vi "Get Displayed Tree Items.vi"(10 "Displayed Items":string[](array[string]), 11 "TreeItems":T1[](array[typedef])) -> (2 "TreeItem Indices (Displayed Items)":i32[](array[numeric]), 3 "TreeItems (duplicate)":T1[](array[typedef]))   [LabVIEW 2020, in "BetterDragAndDrop.lvlib" / "BetterTreeHandle.lvclass"]
uses:
  Classes/BetterTreeHandle/BetterTreeHandle.lvclass
  Classes/BetterTreeItem/SubVIs/TreeItem.ctl
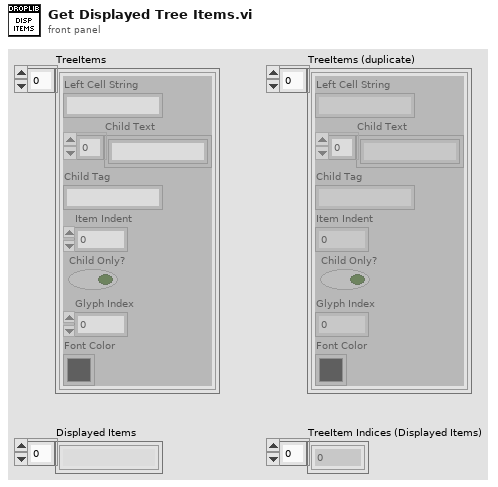
[diagram p1: front panel]
types:
  T1 = typedef "BetterDragAndDrop.lvlib/BetterTreeHandle.lvclass/TreeItem.ctl" = cluster{"Left Cell String":string, "Child Text":string[], "Child Tag":string, "Item Indent":i32, "Child Only?":bool, "Glyph Index":i32, "Font Color":u32}
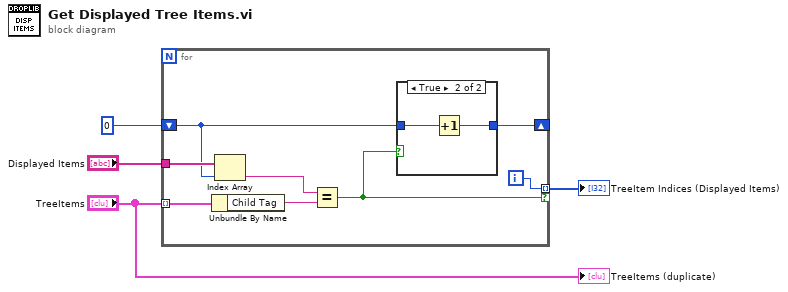
[diagram p0: block diagram]
diagram:
  n1 = for {
    tunnel: "Displayed Items" -> [w11]
    tunnel: [w5] -> w1 mode=indexing if=w8
    tunnel: "TreeItems" -> [w12] mode=indexing
    shift-right: [w6] -> _
    shift-left: 0 -> [w7]
    i -> [w5]
    n2 = Unbundle By Name(w12) -> ("Child Tag"=w10:string)
    n3 = Index Array(array=w11, index=w7) -> (element=w9:string)
    n4 = Equal?(x=w9, y=w10) -> (x = y?=w8:bool)
    n5 = case shown="True" w8 {
      tunnel: w7 -> [w13 w15]
      tunnel: [w13 w14] -> w6
      frame False {
      }
      frame True {
        n6 = Increment(x=w15) -> (x+1=w14:i32)
      }
    }
  }
  "TreeItem Indices (Displayed Items)" <- w1
  "TreeItems (duplicate)" <- "TreeItems"
